vi "Counter - Read Pulse Width and Frequency (On Demand).vi"() -> ()   [LabVIEW 2022 SP3]
doc: "This example demonstrates how to measure period, frequency, pulse width, or two edge separation.\n\nThis example does not use buffering. Since the initiation of the measurement comes from software, it is possible to not acquire every single period of your input signal. To ensure acquisition of every period of your input, you should use Implicit Timing (refer to the other counter input examples).\n\nFor instructions on how to connect your signals to the DAQ device, refer to your device documentation."
uses:
  <vilib>/Utility/error.llb/DialogType.ctl
  <vilib>/DAQmx/read.llb/DAQmx Read (Counter DBL 1Chan 1Samp).vi
  <vilib>/DAQmx/create/channels.llb/DAQmx Create Channel (CI-Period).vi
  <vilib>/DAQmx/create/channels.llb/DAQmx Create Channel (CI-Frequency).vi
  <vilib>/DAQmx/create/channels.llb/DAQmx Create Channel (CI-Pulse Width).vi
  <vilib>/DAQmx/create/channels.llb/DAQmx Create Channel (CI-Two Edge Separation).vi
  <vilib>/DAQmx/miscellaneous.llb/DAQmx Fill In Error Info.vi
  <resource>/objmgr/daqmx.rc
panel:
  in  "Stop":bool
  out "Data":dbl
  in  "Counter Input Type":T1(tab)
  in  "Period Input Terminal":tag="/Dev1/PFI9"
  in  "Max Period":dbl=0.1 format="%0.6f"
  in  "Min Period":dbl=1e-06 format="%0.6f"
  in  "Min Frequency":dbl=2.0 format="%0.6f"
  in  "Max Frequency":dbl=100.0 format="%0.6f"
  in  "Frequency Input Terminal":tag="/Dev1/PFI9"
  in  "Pulse Width Input Terminal":tag="/Dev1/PFI9"
  in  "Min Pulse Width":dbl=1e-06 format="%0.6f"
  in  "Max Pulse Width":dbl=0.1 format="%0.6f"
  in  "Second Input Terminal":tag="/Dev1/PFI9"
  in  "Frst Input Terminal":tag="/Dev1/PFI10"
  in  "Min Separation Time":dbl=1e-06 format="%0.6f"
  in  "Max Separation Time":dbl=0.1 format="%0.6f"
  in  "Counter":tag="Dev1/ctr0"
  # "Channel Settings"
  # "Acquired Data"
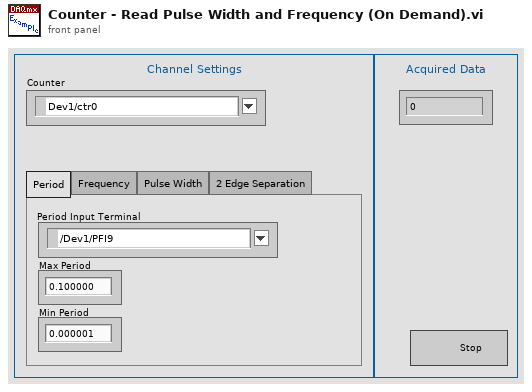
[diagram p1: front panel]
types:
  T1 = enum32{"Period", "Frequency", "Pulse Width", "2 Edge Separation"}
  T2 = typedef "DialogType.ctl" = u16
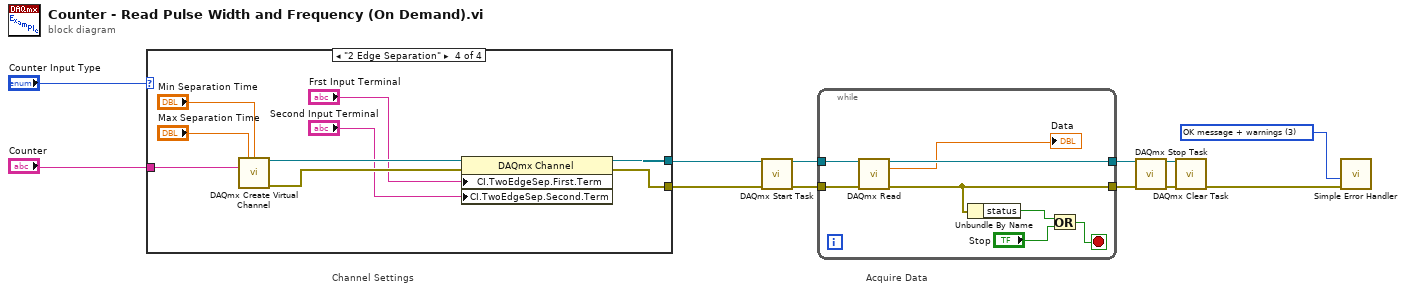
[diagram p0: block diagram]
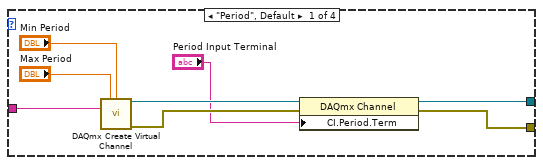
[diagram p2: hidden frame]
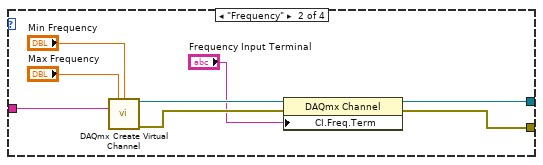
[diagram p3: hidden frame]
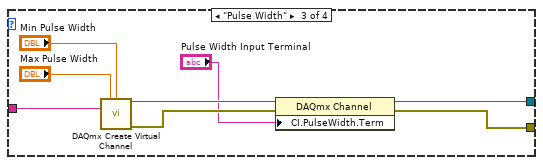
[diagram p4: hidden frame]
diagram:
  w1 = T2 3 items=["no dialog", "OK message", "continue or stop message", "OK message + warnings", "continue/stop + warnings"] ("type of dialog (OK msg:1)")
  # "Acquire Data"
  # "Channel Settings"
  n1 = case shown="\"2 Edge Separation\"" "Counter Input Type" {
    tunnel: [w18 w26 w34 w43] -> w7
    tunnel: [w19 w27 w35 w44] -> w6
    tunnel: "Counter" -> [w20 w28 w36 w45]
    frame "Period", Default {
      n2 = call-poly <vilib>:"DAQmx Create Virtual Channel.vi"("maximum value"="Max Period", "minimum value"="Min Period", "counter"=w20) -> ("task out"=w17:refnum<k21>, "error out"=w16:errorcluster)  [unwired: 11 in]
      n3 = property class="DAQmx Channel"(reference=w17, error in=w16, "CI.Period.Term"="Period Input Terminal") -> (reference out=w19:refnum<k21>, error out=w18:errorcluster)
    }
    frame "Frequency" {
      n4 = call-poly <vilib>:"DAQmx Create Virtual Channel.vi"("maximum value"="Max Frequency", "minimum value"="Min Frequency", "counter"=w28) -> ("task out"=w25:refnum<k21>, "error out"=w24:errorcluster)  [unwired: 11 in]
      n5 = property class="DAQmx Channel"(reference=w25, error in=w24, "CI.Freq.Term"="Frequency Input Terminal") -> (reference out=w27:refnum<k21>, error out=w26:errorcluster)
    }
    frame "Pulse Width" {
      n6 = call-poly <vilib>:"DAQmx Create Virtual Channel.vi"("maximum value"="Max Pulse Width", "minimum value"="Min Pulse Width", "counter"=w36) -> ("task out"=w33:refnum<k21>, "error out"=w32:errorcluster)  [unwired: 11 in]
      n7 = property class="DAQmx Channel"(reference=w33, error in=w32, "CI.PulseWidth.Term"="Pulse Width Input Terminal") -> (reference out=w35:refnum<k21>, error out=w34:errorcluster)
    }
    frame "2 Edge Separation" {
      n8 = call-poly <vilib>:"DAQmx Create Virtual Channel.vi"("maximum value"="Max Separation Time", "minimum value"="Min Separation Time", "counter"=w45) -> ("task out"=w42:refnum<k21>, "error out"=w41:errorcluster)  [unwired: 11 in]
      n9 = property class="DAQmx Channel"(reference=w42, error in=w41, "CI.TwoEdgeSep.First.Term"="Frst Input Terminal", "CI.TwoEdgeSep.Second.Term"="Second Input Terminal") -> (reference out=w44:refnum<k21>, error out=w43:errorcluster)
    }
  }
  n10 = call <vilib>:"DAQmx Start Task.vi"("task/channels in"=w6, "error in"=w7) -> ("task out"=w12:refnum<k21>, "error out"=w11:errorcluster)  [unwired: 12 in]
  n11 = while {
    tunnel: w12 -> [w53]
    tunnel: w11 -> [w52]
    tunnel: [w51] -> w2
    tunnel: [w49] -> w3
    stop <- w46 stop-if-true
    n12 = call-poly <vilib>:"DAQmx Read.vi"("task/channels in"=w53, "error in"=w52) -> ("task out"=w51:refnum<k21>, "data"=→"Data":dbl, "error out"=w49:errorcluster)  [unwired: 11 in]
    n13 = Unbundle By Name(w49) -> ("status"=w48:bool)
    n14 = Or(x=w48, y="Stop") -> (x .or. y?=w46:bool)
  }
  n15 = call <vilib>:"DAQmx Stop Task.vi"("task/channels in"=w2, "error in"=w3) -> ("task out"=w5:refnum<k21>, "error out"=w4:errorcluster)  [unwired: 12 in]
  n16 = call <vilib>:"DAQmx Clear Task.vi"("task in"=w5, "error in"=w4) -> ("error out"=w10:errorcluster)  [unwired: 13 in]
  n17 = call <vilib>:"Simple Error Handler.vi"("type of dialog (OK msg:1)"=w1, "error in (no error)"=w10) -> ()  [unwired: 3 in, 5 out]
